vi "PinMapService QueryRelays.vi"(6 "contextId":T1, 8 "error in":errorcluster, 9 "timeout (ms)":i32=-1, 10 "Request Data":T5, 11 "gRPC ID":T1) -> (0 "error out":errorcluster, 2 "Response Data":T2, 3 "gRPC ID out":T1)   [LabVIEW 2020, in "Measurement Plugin Pin Map Client.lvlib"]
uses:
  Measurement Plugin Pin Map Client.lvlib
  <vilib>/gRPC/LabVIEW gRPC Library/Shared/grpcId.ctl
  RPC Messages/ni_measurementlink_pinmap_v1_QueryRelaysRequest.ctl
  RPC Messages/ni_measurementlink_pinmap_v1_QueryRelaysResponse.ctl
  RPC Messages/ni_measurementlink_pinmap_v1_RelayDefinition.ctl
  RPC Messages/ni_measurementlink_pinmap_v1_RelayGroupDefinition.ctl
  RPC Messages/ni_measurementlink_pinmap_v1_QueryRelaysResponse_Flat.ctl
  RPC Messages/ni_measurementlink_pinmap_v1_RelayDefinition_Flat.ctl
  RPC Messages/ni_measurementlink_pinmap_v1_RelayGroupDefinition_Flat.ctl
  14035477-4c25-4107-8ed5-d0c4ef420ce5.vi
  <vilib>/gRPC/LabVIEW gRPC Library/Shared/TranslateGrpcError.vi
  <vilib>/gRPC/LabVIEW gRPC Library/Shared/Wait On Occurence.vi
  RPC Messages/FlatToRichni_measurementlink_pinmap_v1_RelayDefinition.vi
  RPC Messages/FlatToRichni_measurementlink_pinmap_v1_RelayGroupDefinition.vi
  <vilib>/gRPC/LabVIEW gRPC Library/Server API/Server/Get Server DLL Path.vi
  <vilib>/Utility/error.llb/Error Cluster From Error Code.vi
  <vilib>/Utility/error.llb/Simple Error Handler.vi
  <vilib>/gRPC/LabVIEW gRPC Library/grpc-lvsupport-release.lvlib
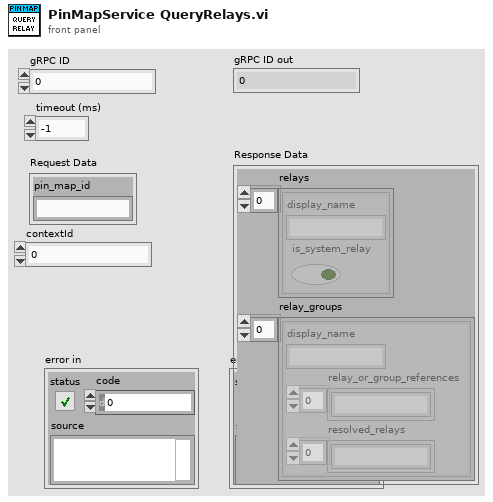
[diagram p1: front panel]
types:
  T1 = typedef "grpc-lvsupport-release.lvlib/grpcId.ctl" = u64
  T2 = typedef "Measurement Plugin Pin Map Client.lvlib/ni_measurementlink_pinmap_v1_QueryRelaysResponse.ctl" = cluster{"relays":T3[], "relay_groups":T4[]}
  T3 = typedef "Measurement Plugin Pin Map Client.lvlib/ni_measurementlink_pinmap_v1_RelayDefinition.ctl" = cluster{"display_name":string, "is_system_relay":bool}
  T4 = typedef "Measurement Plugin Pin Map Client.lvlib/ni_measurementlink_pinmap_v1_RelayGroupDefinition.ctl" = cluster{"display_name":string, "relay_or_group_references":string[], "resolved_relays":string[]}
  T5 = typedef "Measurement Plugin Pin Map Client.lvlib/ni_measurementlink_pinmap_v1_QueryRelaysRequest.ctl" = cluster{"pin_map_id":string}
  T6 = typedef "Measurement Plugin Pin Map Client.lvlib/ni_measurementlink_pinmap_v1_QueryRelaysResponse_Flat.ctl" = cluster{"relays":T7[], "relay_groups":T8[]}
  T7 = typedef "Measurement Plugin Pin Map Client.lvlib/ni_measurementlink_pinmap_v1_RelayDefinition_Flat.ctl" = cluster{"display_name":string, "is_system_relay":bool}
  T8 = typedef "Measurement Plugin Pin Map Client.lvlib/ni_measurementlink_pinmap_v1_RelayGroupDefinition_Flat.ctl" = cluster{"display_name":string, "relay_or_group_references":string[], "resolved_relays":string[]}
  T9 = typedef "Measurement Plugin Pin Map Client.lvlib/ni_measurementlink_pinmap_v1_QueryRelaysRequest_Flat.ctl" = cluster{"pin_map_id":string}
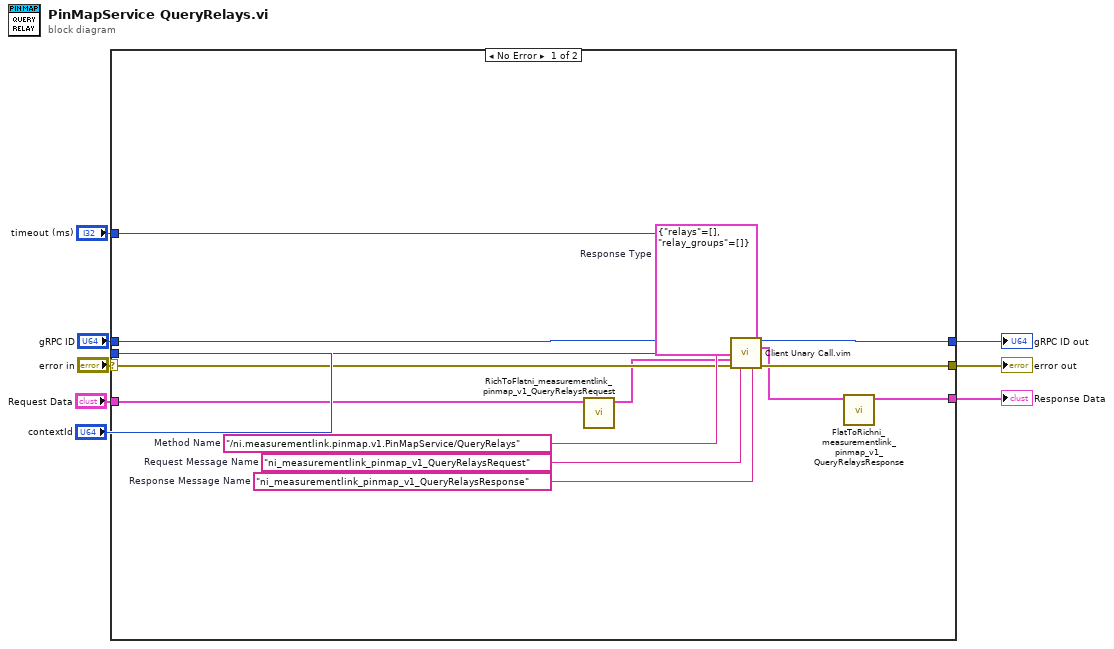
[diagram p0: block diagram]
diagram:
  n1 = case shown="No Error" "error in" {
    selector: "error in" -> [w18 w23]
    tunnel: [w17 w23] -> w7
    tunnel: "gRPC ID" -> [w16 w24]
    tunnel: [w15 w24] -> w5
    tunnel: "Request Data" -> [w12 _]
    tunnel: [w9 _] -> w3
    tunnel: "timeout (ms)" -> [w14 _]
    tunnel: "contextId" -> [w13 _]
    frame No Error {
      w19 = "ni_measurementlink_pinmap_v1_QueryRelaysResponse"  # Response Message Name
      w20 = "ni_measurementlink_pinmap_v1_QueryRelaysRequest"  # Request Message Name
      w21 = T6 {"relays"=[], "relay_groups"=[]}  # Response Type
      w22 = "/ni.measurementlink.pinmap.v1.PinMapService/QueryRelays"  # Method Name
      n2 = call "RichToFlatni_measurementlink_pinmap_v1_QueryRelaysRequest.vi"("InputCluster"=w12) -> ("OutputCluster"=w11:T9)  [unwired: 10 in]
      n3 = call "Client Unary Call.vim"("ClientID in"=w16, "Response Type"=w21, "timeout (ms)"=w14, "Method Name"=w22, "contextId"=w13, "Request Data"=w11, "error in"=w18, "Request Message Name"=w20, "Response Message Name"=w19) -> ("ClientID out"=w15:u64, "Response Data"=w10:T6, "error out"=w17:errorcluster)  [unwired: 4 in]
      n4 = call "FlatToRichni_measurementlink_pinmap_v1_QueryRelaysResponse.vi"("InputCluster"=w10) -> ("OutputCluster"=w9:T2)  [unwired: 10 in]
    }
    frame Error {
    }
  }
  "error out" <- w7
  "gRPC ID out" <- w5
  "Response Data" <- w3
